vi "Operator judge LVDT's TP.vi"(6 "LVDT's Limits":T1[](array[typedef]) {"Lower Limit" format="%.2f"; "Upper Limit" format="%.2f"}, 11 "LVDT's Array":sgl[](array[numeric])) -> ()   [LabVIEW 2018]
uses:
  type defs/EOL LVDT's Check Controller.ctl
panel:
  out "Tank 12":dbl(slide) min=-5.0 max=5.0 scale=-5.0..5.0 scale format="%#_4g"
  out "Tank 11":dbl(slide) min=-5.0 max=5.0 scale=-5.0..5.0 scale format="%#_4g"
  out "Tank 10":dbl(slide) min=-5.0 max=5.0 scale=-5.0..5.0 scale format="%#_4g"
  out "Tank 9":dbl(slide) min=-5.0 max=5.0 scale=-5.0..5.0 scale format="%#_4g"
  out "Tank 8":dbl(slide) min=-5.0 max=5.0 scale=-5.0..5.0 scale format="%#_4g"
  out "Tank 7":dbl(slide) min=-5.0 max=5.0 scale=-5.0..5.0 scale format="%#_4g"
  out "Tank 6":dbl(slide) min=-5.0 max=5.0 scale=-5.0..5.0 scale format="%#_4g"
  out "Tank 5":dbl(slide) min=-5.0 max=5.0 scale=-5.0..5.0 scale format="%#_4g"
  out "Tank 4":dbl(slide) min=-5.0 max=5.0 scale=15.0..25.0 scale format="%#_4g"
  out "Tank 3":dbl(slide) min=-5.0 max=5.0 scale=-10.0..10.0 scale format="%#_4g"
  out "Tank 2":dbl(slide) min=-5.0 max=5.0 scale=-6.0..6.0 scale format="%#_4g"
  out "Tank 1":dbl(slide) min=-5.0 max=5.0 scale=-5.0..5.0 scale format="%#_4g"
  # "X1"
  # "X5"
  # "Z1"
  # "Z5"
  # "Z19"
  # "Z11"
  # "Z25"
  # "Z33"
  # "Z40"
  # "Z44"
  # "X10"
  # "X6"
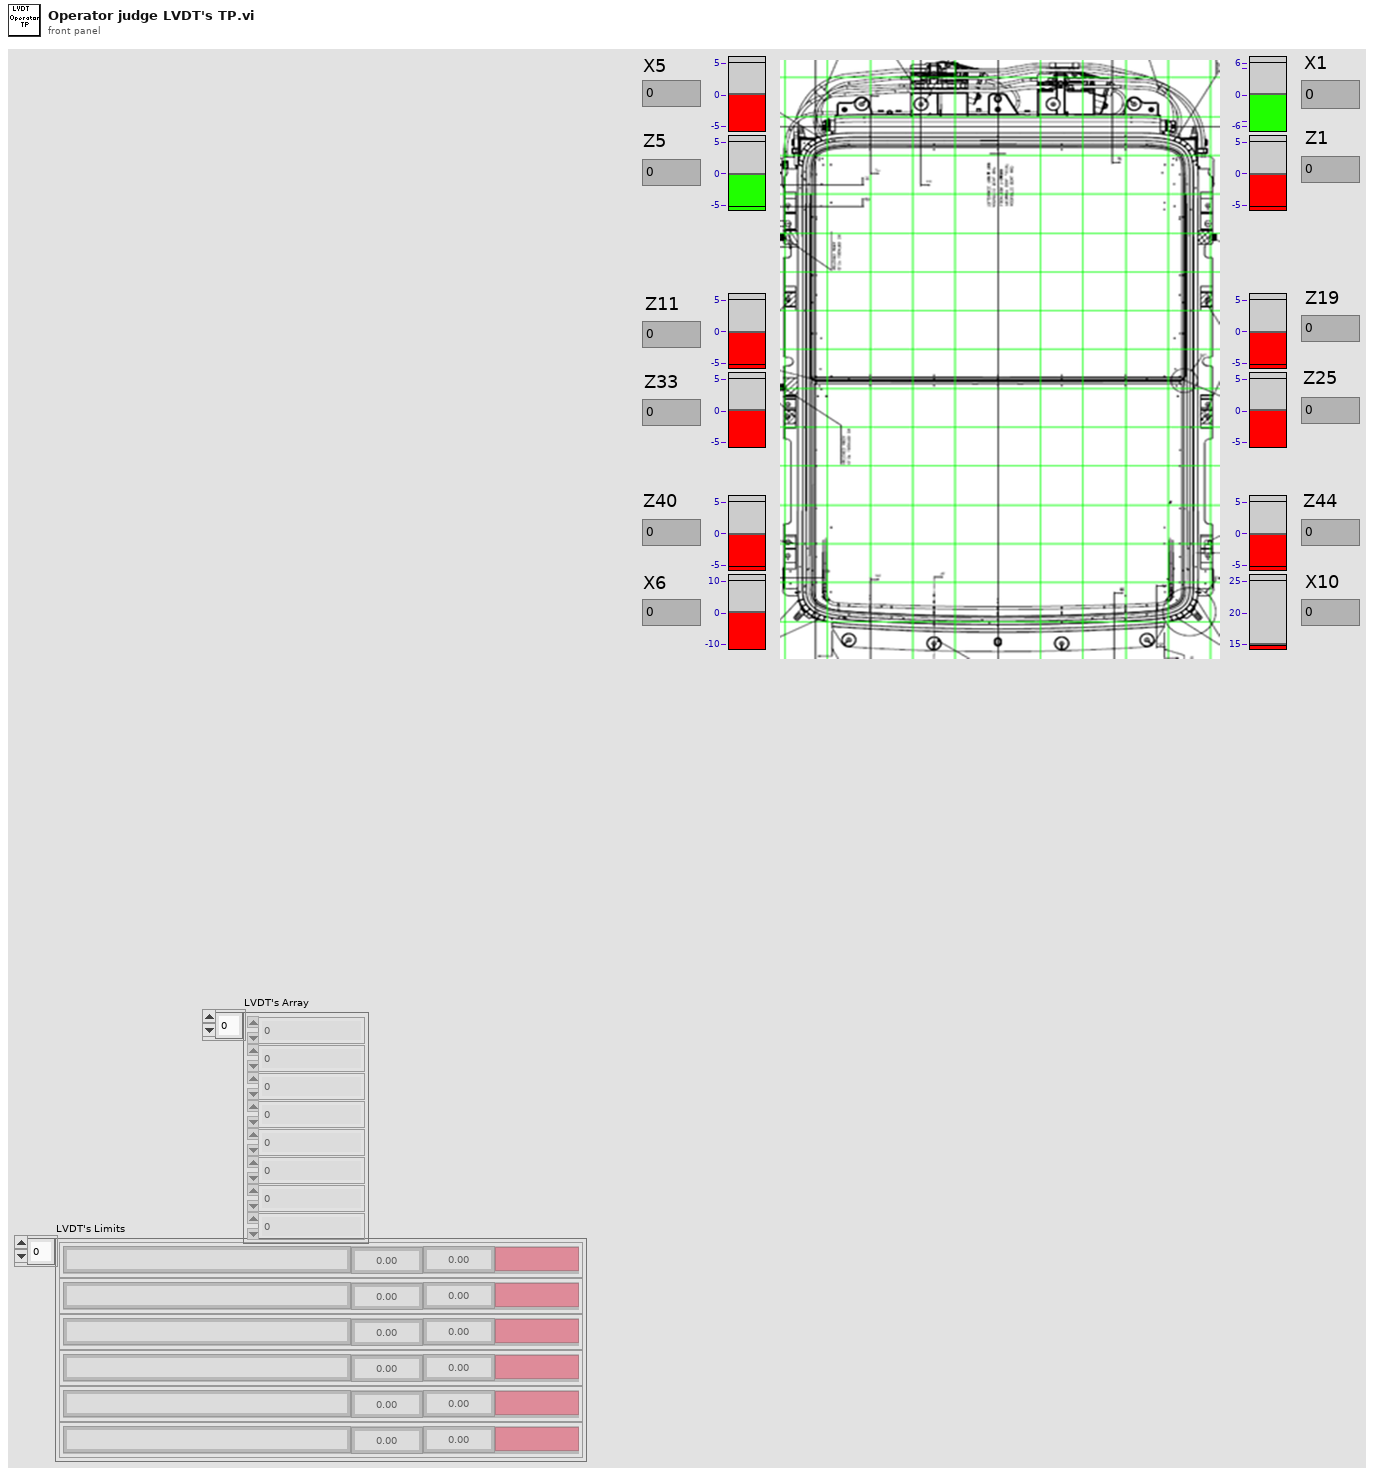
[diagram p1: front panel]
types:
  T1 = typedef "EOL LVDT's Check Controller.ctl" = cluster{"Upper Limit":dbl, "Lower Limit":dbl, "LVDT Name":string, "Check":bool}
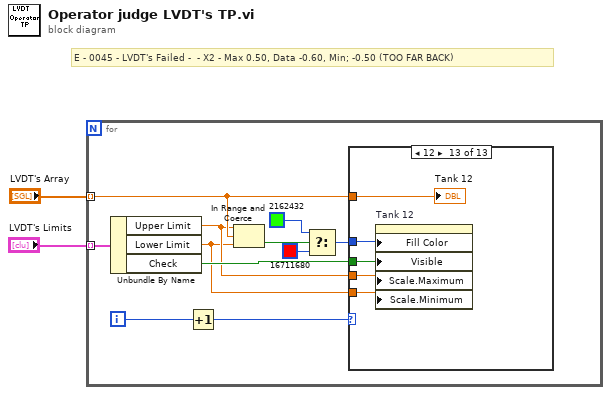
[diagram p0: block diagram]
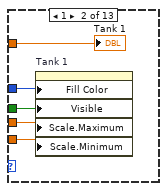
[diagram p3: hidden frame]
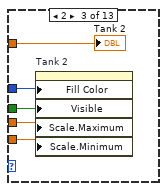
[diagram p4: hidden frame]
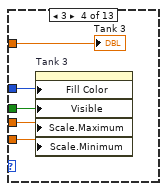
[diagram p5: hidden frame]
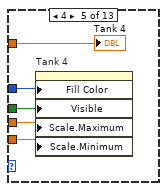
[diagram p6: hidden frame]
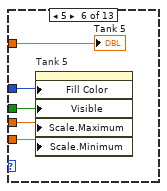
[diagram p7: hidden frame]
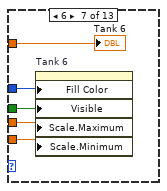
[diagram p8: hidden frame]
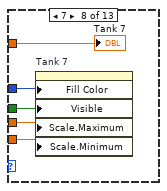
[diagram p9: hidden frame]
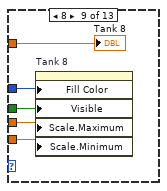
[diagram p10: hidden frame]
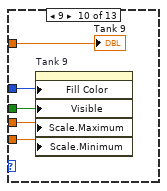
[diagram p11: hidden frame]
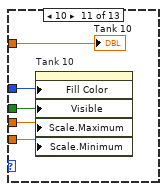
[diagram p12: hidden frame]
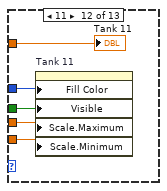
[diagram p13: hidden frame]
diagram:
  # "E - 0045 - LVDT's Failed -  - X2 - Max 0.50, Data -0.60, Min; -0.50 (TOO FAR BACK)"
  n1 = for {
    tunnel: "LVDT's Array" -> [w7] mode=indexing
    tunnel: "LVDT's Limits" -> [w13] mode=indexing
    i -> [w5]
    n2 = Unbundle By Name(w13) -> ("Upper Limit"=w4:dbl, "Lower Limit"=w3:dbl, "Check"=w12:bool)
    n3 = Increment(x=w5) -> (x+1=w6:i32)
    n4 = In Range and Coerce(upper limit=w4, x=w7, lower limit=w3) -> (In Range?=w9:bool)  [unwired: 1 out]
    n5 = Select(t=u32 2162432, s=w9, f=u32 16711680) -> (s? t:f=w8:u32)
    n6 = case shown="12" w6 {
      tunnel: w12 -> [_ w16 w21 w26 w31 w36 w41 w46 w51 w56 w61 w66 w71]
      tunnel: w8 -> [_ w17 w22 w27 w32 w37 w42 w47 w52 w57 w62 w67 w72]
      tunnel: w7 -> [_ w18 w23 w28 w33 w38 w43 w48 w53 w58 w63 w68 w73]
      tunnel: w4 -> [_ w15 w20 w25 w30 w35 w40 w45 w50 w55 w60 w65 w70]
      tunnel: w3 -> [_ w14 w19 w24 w29 w34 w39 w44 w49 w54 w59 w64 w69]
      frame 0, Default {
      }
      frame 1 {
        n7 = property on="Tank 1" class="Slide (严格)"("Fill Color"=w17, "Visible"=w16, "Scale.Maximum"=w15, "Scale.Minimum"=w14) -> ()  [unwired: 2 in, 2 out]
        "Tank 1" <- w18
      }
      frame 2 {
        n8 = property on="Tank 2" class="Slide (严格)"("Fill Color"=w22, "Visible"=w21, "Scale.Maximum"=w20, "Scale.Minimum"=w19) -> ()  [unwired: 2 in, 2 out]
        "Tank 2" <- w23
      }
      frame 3 {
        n9 = property on="Tank 3" class="Slide (严格)"("Fill Color"=w27, "Visible"=w26, "Scale.Maximum"=w25, "Scale.Minimum"=w24) -> ()  [unwired: 2 in, 2 out]
        "Tank 3" <- w28
      }
      frame 4 {
        n10 = property on="Tank 4" class="Slide (严格)"("Fill Color"=w32, "Visible"=w31, "Scale.Maximum"=w30, "Scale.Minimum"=w29) -> ()  [unwired: 2 in, 2 out]
        "Tank 4" <- w33
      }
      frame 5 {
        n11 = property on="Tank 5" class="Slide (严格)"("Fill Color"=w37, "Visible"=w36, "Scale.Maximum"=w35, "Scale.Minimum"=w34) -> ()  [unwired: 2 in, 2 out]
        "Tank 5" <- w38
      }
      frame 6 {
        n12 = property on="Tank 6" class="Slide (严格)"("Fill Color"=w42, "Visible"=w41, "Scale.Maximum"=w40, "Scale.Minimum"=w39) -> ()  [unwired: 2 in, 2 out]
        "Tank 6" <- w43
      }
      frame 7 {
        n13 = property on="Tank 7" class="Slide (严格)"("Fill Color"=w47, "Visible"=w46, "Scale.Maximum"=w45, "Scale.Minimum"=w44) -> ()  [unwired: 2 in, 2 out]
        "Tank 7" <- w48
      }
      frame 8 {
        n14 = property on="Tank 8" class="Slide (严格)"("Fill Color"=w52, "Visible"=w51, "Scale.Maximum"=w50, "Scale.Minimum"=w49) -> ()  [unwired: 2 in, 2 out]
        "Tank 8" <- w53
      }
      frame 9 {
        n15 = property on="Tank 9" class="Slide (严格)"("Fill Color"=w57, "Visible"=w56, "Scale.Maximum"=w55, "Scale.Minimum"=w54) -> ()  [unwired: 2 in, 2 out]
        "Tank 9" <- w58
      }
      frame 10 {
        n16 = property on="Tank 10" class="Slide (严格)"("Fill Color"=w62, "Visible"=w61, "Scale.Maximum"=w60, "Scale.Minimum"=w59) -> ()  [unwired: 2 in, 2 out]
        "Tank 10" <- w63
      }
      frame 11 {
        n17 = property on="Tank 11" class="Slide (严格)"("Fill Color"=w67, "Visible"=w66, "Scale.Maximum"=w65, "Scale.Minimum"=w64) -> ()  [unwired: 2 in, 2 out]
        "Tank 11" <- w68
      }
      frame 12 {
        n18 = property on="Tank 12" class="Slide (严格)"("Fill Color"=w72, "Visible"=w71, "Scale.Maximum"=w70, "Scale.Minimum"=w69) -> ()  [unwired: 2 in, 2 out]
        "Tank 12" <- w73
      }
    }
  }
